vi "refreash peaks.vi"(7 "element":cluster{"Locations":dbl[], "Amplitudes":dbl[]}, 8 "error in":errorcluster, 9 "List Parameter Fit in":dbl[][](array[numeric]), 10 "List ROI in":dbl[][](array[numeric]), 11 "Spectrum":refnum<vi>) -> (0 "error out":errorcluster, 1 "List Parameter Fit Out":dbl[][](array[numeric]), 2 "List ROI Out":dbl[][](array[numeric]), 3 "Peaks Out":cluster{"Locations":dbl[], "Amplitudes":dbl[]}, 4 "Table":string[][](table))   [LabVIEW 2023]
uses:
  bbd1353a-11db-48cb-8e6e-7bc43c4b74a2.vi
  c29d4322-1a4b-4959-84e7-67fa9e6d6261.vi
  e8004514-cfb5-4b90-ae77-451f506fadd8.vi
  <vilib>/Utility/Data Type/Get Array Information.vi
  <vilib>/Utility/Data Type/Get Type Information.vi
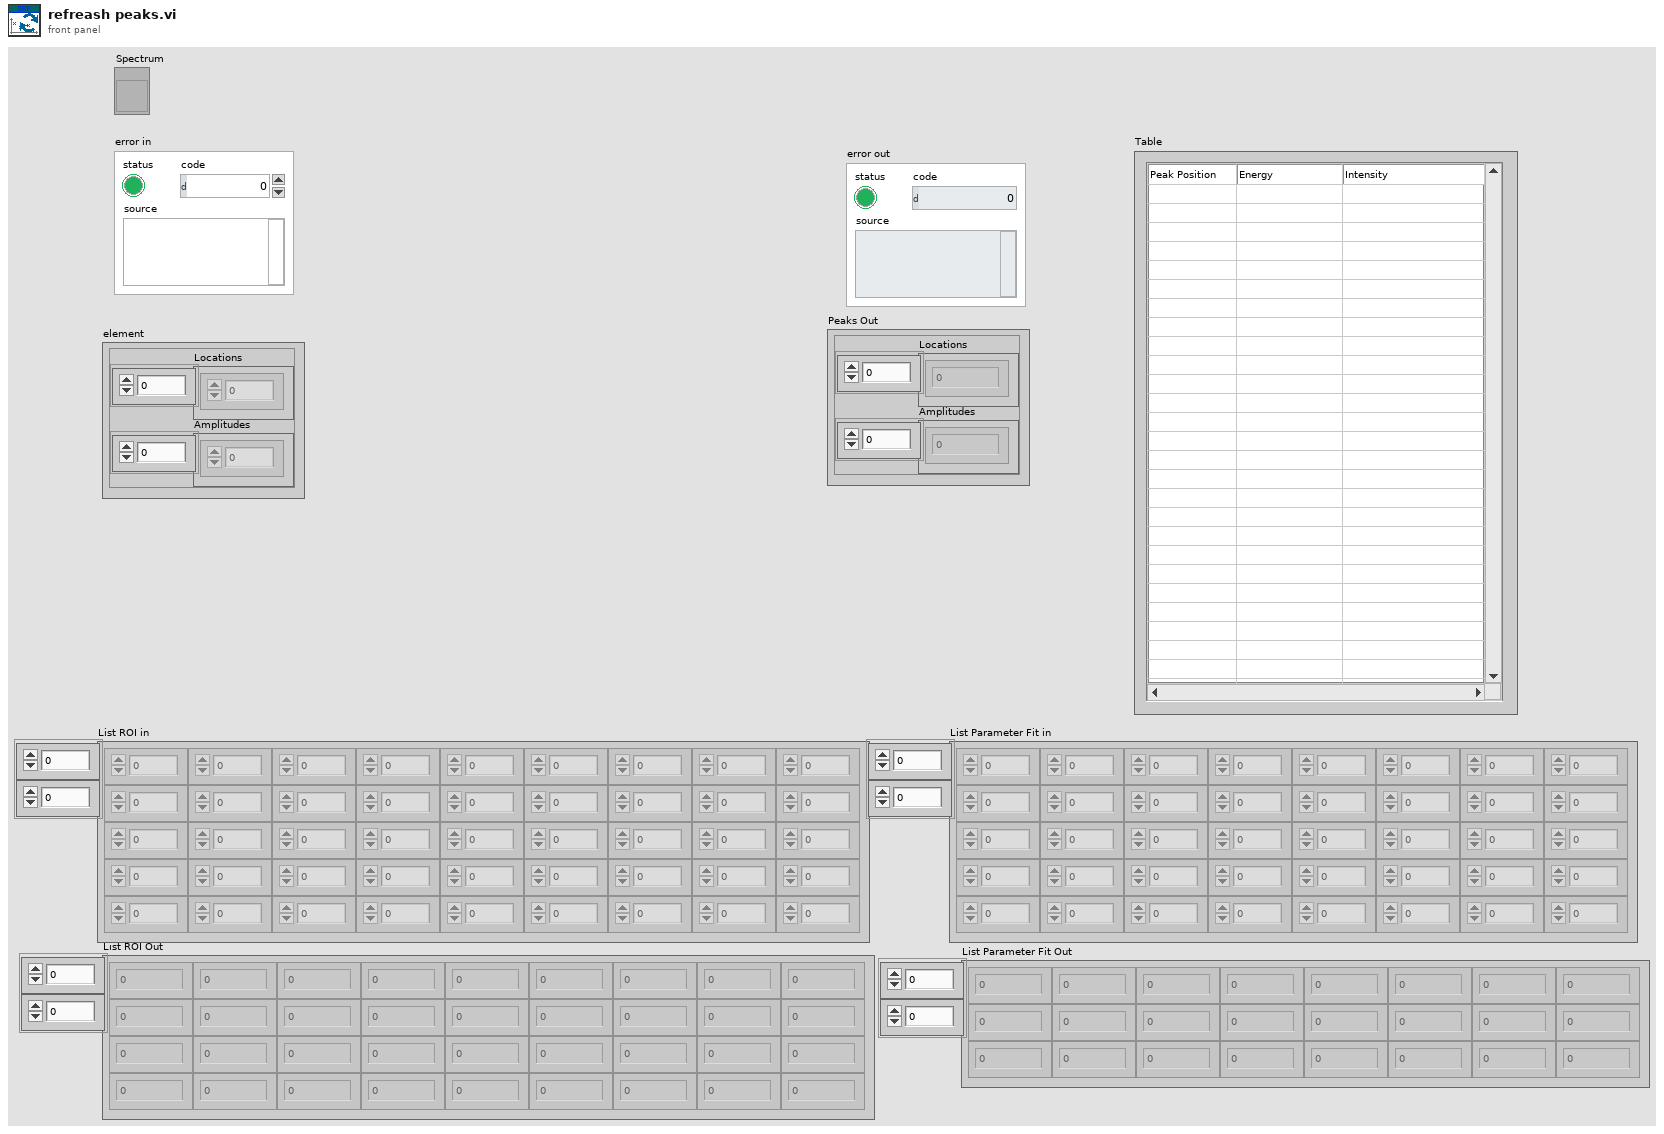
[diagram p1: front panel]
types:
  T1 = typedef "LVCursorListTypeDef.ctl" = cluster{"Name":string, "Color":u32, "Style":u8, "Point Style":u8, "Name Visible":bool, "Allow Drag":bool, "Cursor Mode":u32, "Plot":i32, "Index":i32, "Position":cluster{"X":dbl, "Y":dbl}, "X Scale":u32, "Y Scale":u32, "Watch Plots":i32[], "Watch All Plots":bool, "Plot Area":i32, "Label Offset":cluster{"X":dbl, "Y":dbl}}[]
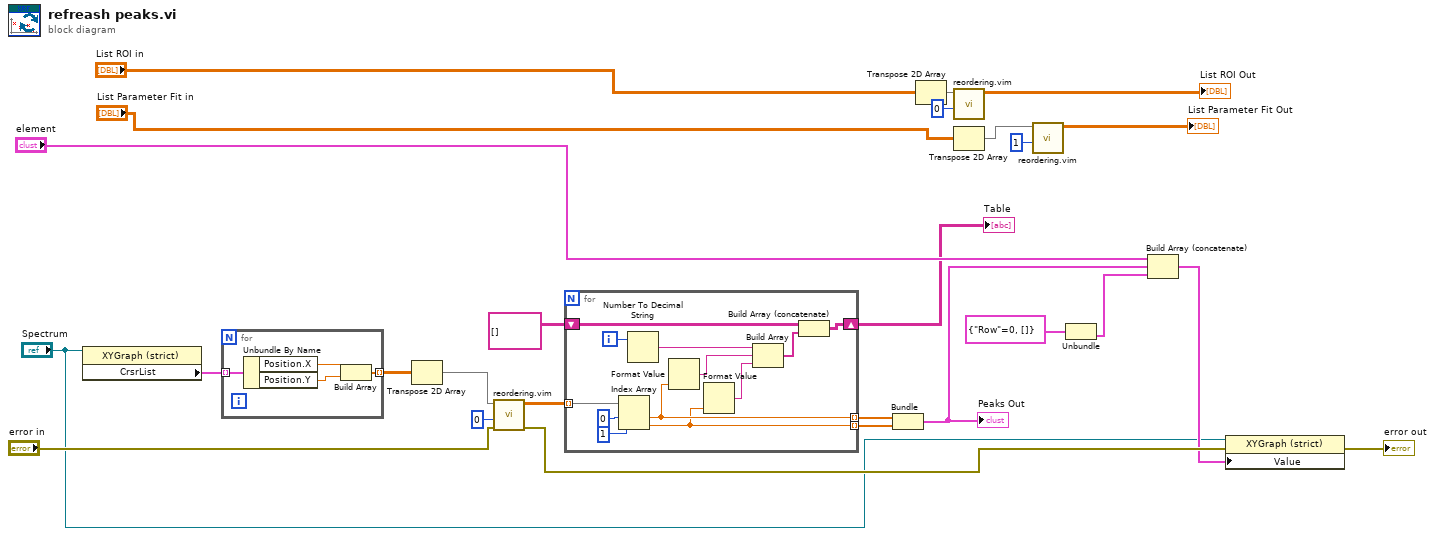
[diagram p0: block diagram]
diagram:
  n1 = property on="Property Node" class="XYGraph (strict)"(reference="Spectrum") -> ("CrsrList"=w18:T1)  [unwired: 1 in, 2 out]
  n2 = for {
    tunnel: w18 -> [w30] mode=indexing
    tunnel: [w27] -> w25 mode=indexing
    n3 = Unbundle By Name(w30) -> ("Position.X"=w29:dbl, "Position.Y"=w28:dbl)
    n4 = Build Array(w29, w28) -> (w27:dbl[])
  }
  n5 = Transpose 2D Array(2D array=w25) -> (transposed array=w24:dbl[][])
  n6 = call "reordering.vim"("error in (no error)"="error in", "Row to Reorder"=0, "Data In"=w24) -> ("Error Out"=w16:errorcluster, "Data Out"=w22:dbl[][])  [unwired: 7 in]
  n7 = for {
    tunnel: w22 -> [w42] mode=indexing
    tunnel: [w38] -> w20 mode=indexing
    tunnel: [w37] -> w19 mode=indexing
    shift-right: [w31] -> w9
    shift-left: string[][] [] ("Table") -> [w33]
    i -> [w39]
    n8 = Index Array(array=w42, index #1=0 ("index"), index #2=1 ("index")) -> (element #1=w38:dbl, element #2=w37:dbl)
    n9 = Number To Decimal String(number=w39) -> (decimal integer string=w34:string)  [unwired: 1 in]
    n10 = Format Value(value (0)=w38) -> (output string=w35:string)  [unwired: 2 in]
    n11 = Format Value(value (0)=w37) -> (output string=w36:string)  [unwired: 2 in]
    n12 = Build Array(w34, w35, w36) -> (w32:string[])
    n13 = Build Array (concatenate)(w33, w32) -> (w31:string[][])
  }
  "Table" <- w9
  n14 = Bundle(w20, w19) -> (w12:cluster{dbl[], dbl[]})  [unwired: 1 in]
  "Peaks Out" <- w12
  n15 = Transpose 2D Array(2D array="List ROI in") -> (transposed array=w8:dbl[][])
  n16 = call "reordering.vim"("Row to Reorder"=0, "Data In"=w8) -> ("Data Out"=→"List ROI Out":dbl[][])  [unwired: 8 in, 1 out]
  n17 = Transpose 2D Array(2D array="List Parameter Fit in") -> (transposed array=w6:dbl[][])
  n18 = call "reordering.vim"("Row to Reorder"=1, "Data In"=w6) -> ("Data Out"=→"List Parameter Fit Out":dbl[][])  [unwired: 8 in, 1 out]
  n19 = Unbundle(cluster{"Row":i32, cluster{dbl[], dbl[]}[]} {"Row"=0, []}) -> (w13:cluster{dbl[], dbl[]}[])  [unwired: 1 out]
  n20 = Build Array (concatenate)("element", w12, w13) -> (w11:cluster{"Locations":dbl[], "Amplitudes":dbl[]}[])
  n21 = property on="Property Node" class="XYGraph (strict)"(reference="Spectrum", error in=w16, "Value"=w11) -> (error out=→"error out":errorcluster)  [unwired: 1 out]
